vi "Close thermocouple VI.vi"(8 "error in (no error)":errorcluster) -> (0 "error out":errorcluster)   [LabVIEW 2019]
panel:
  out "msg_subsys":string
  out "format string":string
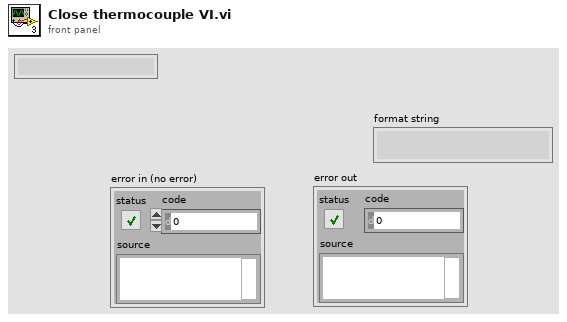
[diagram p1: front panel]
types:
  T1 = enum32{"Bad", "Idle", "Run top level", "Running"}
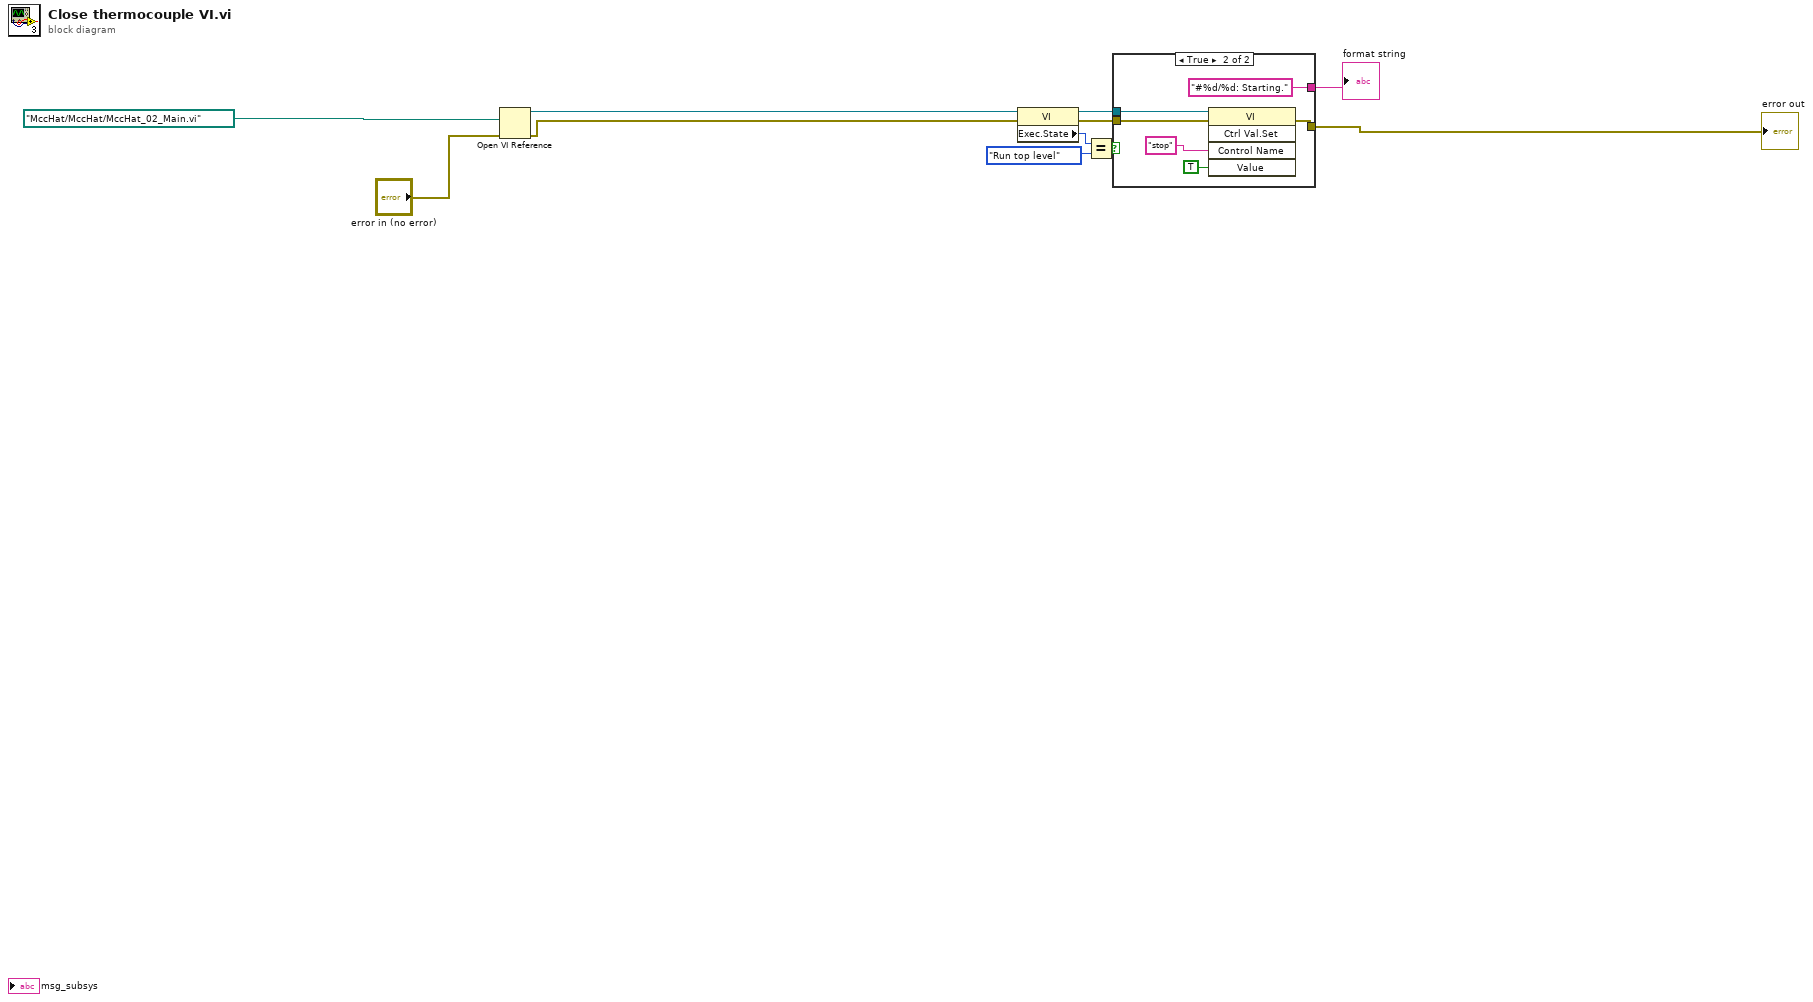
[diagram p0: block diagram]
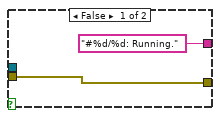
[diagram p2: hidden frame]
diagram:
  n1 = Open VI Reference(vi path=path "MccHat/MccHat/MccHat_02_Main.vi", error in (no error)="error in (no error)") -> (vi reference=w7:refnum<vi>, error out=w11:errorcluster)  [unwired: 4 in]
  n2 = property class="VI"(reference=w7, error in=w11) -> (reference out=w6:refnum<vi>, error out=w5:errorcluster, "Exec.State"=w4:T1)
  n3 = Equal?(x=w4, y=T1."Run top level" ("Execution:State")) -> (x = y?=w2:bool)
  n4 = case shown="True" w2 {
    tunnel: w6 -> [_ w18]
    tunnel: w5 -> [w13 w17]
    tunnel: [w13 w16] -> w8
    tunnel: ["#%d/%d: Running." ("format string") "#%d/%d: Starting." ("format string")] -> w1
    frame False {
    }
    frame True {
      n5 = invoke class="VI" method="Ctrl Val.Set"(reference=w18, error in=w17, "Control Name"="stop", "Value"=TRUE ("Auto Dispose Reference")) -> (error out=w16:errorcluster)  [unwired: 1 in, 4 out]
    }
  }
  "error out" <- w8
  "format string" <- w1
